vi "时间解析.vi"() -> (0 "数组":string[](array[string]))   [LabVIEW 2015]
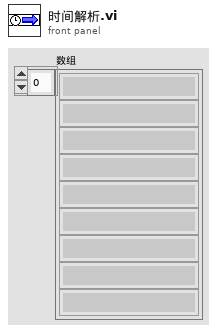
[diagram p1: front panel]
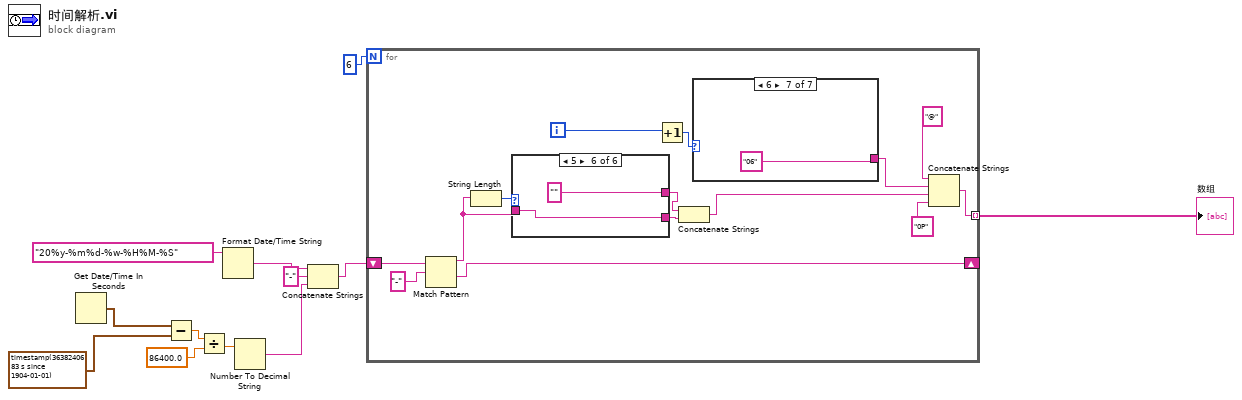
[diagram p0: block diagram]
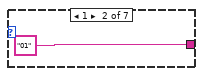
[diagram p3: hidden frame]
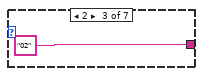
[diagram p4: hidden frame]
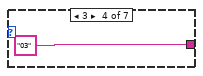
[diagram p5: hidden frame]
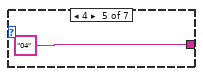
[diagram p6: hidden frame]
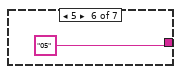
[diagram p7: hidden frame]
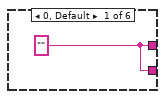
[diagram p8: hidden frame]
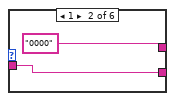
[diagram p9: hidden frame]
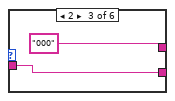
[diagram p10: hidden frame]
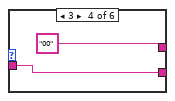
[diagram p11: hidden frame]
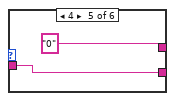
[diagram p12: hidden frame]
diagram:
  n1 = Get Date/Time In Seconds() -> (seconds since 1Jan1904=w9:timestamp)
  n2 = Subtract(x=w9, y=timestamp(3638240683.009 s since 1904-01-01) ("时间标识")) -> (x-y=w7:dbl)
  n3 = Divide(x=w7, y=86400.0) -> (x/y=w5:dbl)
  n4 = Format Date/Time String(time format string (%c)="20%y-%m%d-%w-%H%M-%S" ("时间格式字符串(%c)")) -> (date/time string=w4:string)  [unwired: 2 in]
  n5 = Number To Decimal String(number=w5) -> (decimal integer string=w2:string)  [unwired: 1 in]
  n6 = Concatenate Strings(w4, "-" ("字符串"), w2) -> (w1:string)
  n7 = for {
    N: 6 -> [_]
    shift-right: [w24] -> _
    shift-left: w1 -> [w25]
    tunnel: [w19] -> w10 mode=indexing
    i -> [w14]
    n8 = Match Pattern(string=w25, regular expression="-" ("正则表达式")) -> (before substring=w22:string, after substring=w24:string)  [unwired: 1 in, 2 out]
    n9 = String Length(string=w22) -> (length=w23:i32)
    n10 = case shown="5" w23 {
      tunnel: w22 -> [_ w35 w37 w39 w41 w43]
      tunnel: [w33 "0000" ("正则表达式") "000" ("正则表达式") "00" ("正则表达式") "0" ("正则表达式") "" ("正则表达式")] -> w21
      tunnel: [w33 w35 w37 w39 w41 w43] -> w20
      frame 0, Default {
        w33 = "" ("正则表达式")
      }
      frame 1 {
      }
      frame 2 {
      }
      frame 3 {
      }
      frame 4 {
      }
      frame 5 {
      }
    }
    n11 = Increment(x=w14) -> (x+1=w13:i32)
    n12 = Concatenate Strings(w21, w20) -> (w18:string)
    n13 = case shown="6" w13 {
      tunnel: [_ "01" ("字符串") "02" ("字符串") "03" ("字符串") "04" ("字符串") "05" ("字符串") "06" ("字符串")] -> w15
      frame 0, Default {
      }
      frame 1 {
      }
      frame 2 {
      }
      frame 3 {
      }
      frame 4 {
      }
      frame 5 {
      }
      frame 6 {
      }
    }
    n14 = Concatenate Strings("@" ("字符串"), w15, w18, "0P" ("字符串")) -> (w19:string)
  }
  "数组" <- w10
